vi "ABB Select pages.vi"(7 "Page Names":string[](array[string]), 9 "Report in":string, 10 "Page ends":i32[](array[numeric]), 11 "Page select":bool[](array[boolean])) -> (1 "Report out":string, 2 "Page names out":string[](array[string]), 4 "Pages out":string[](array[string]))   [LabVIEW 2017]
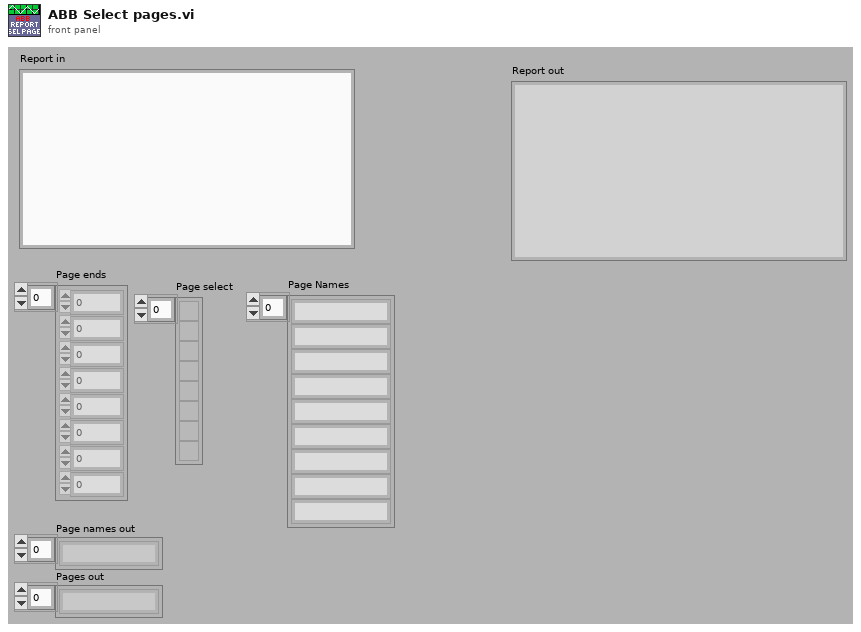
[diagram p1: front panel]
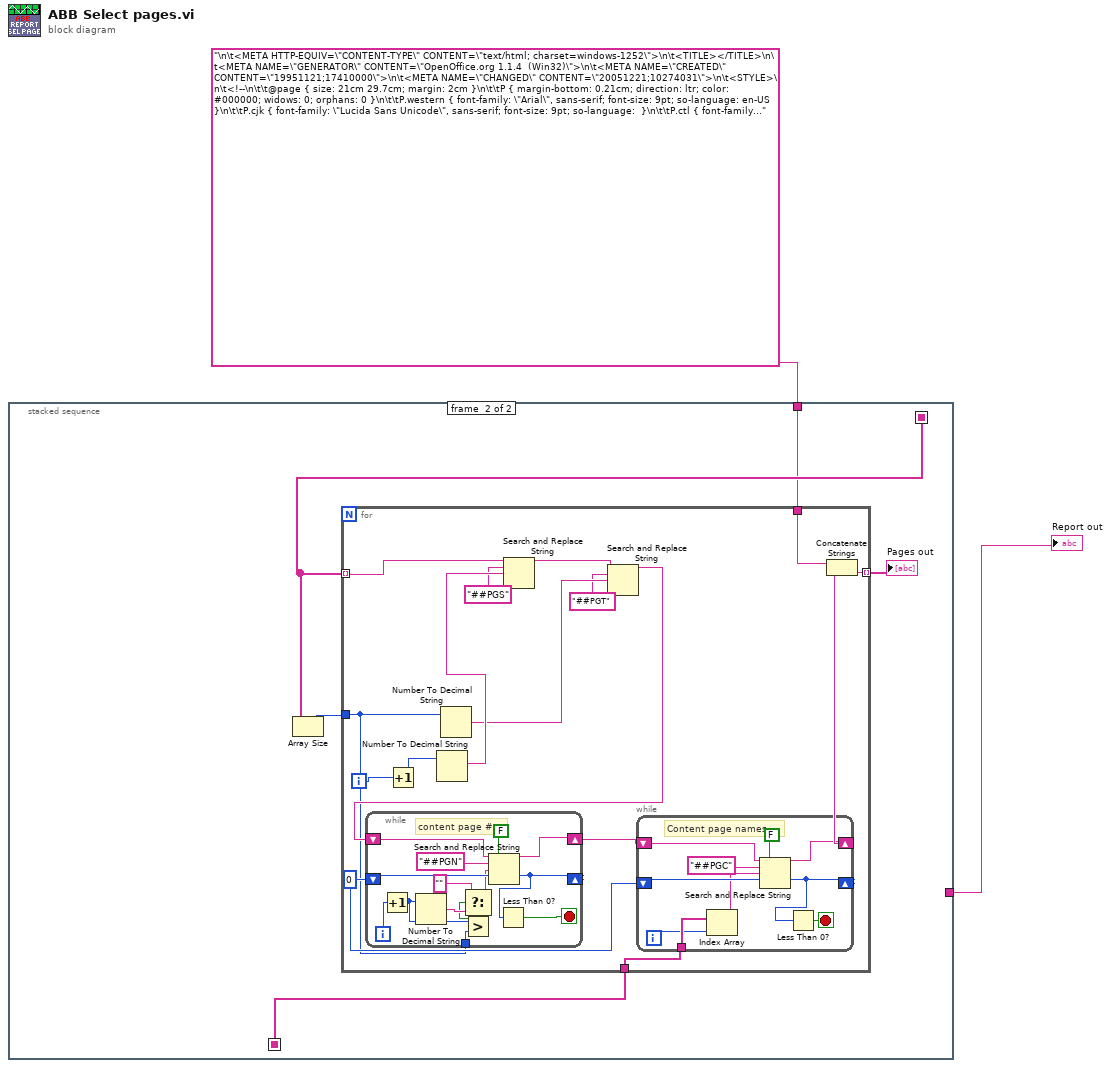
[diagram p0: block diagram]
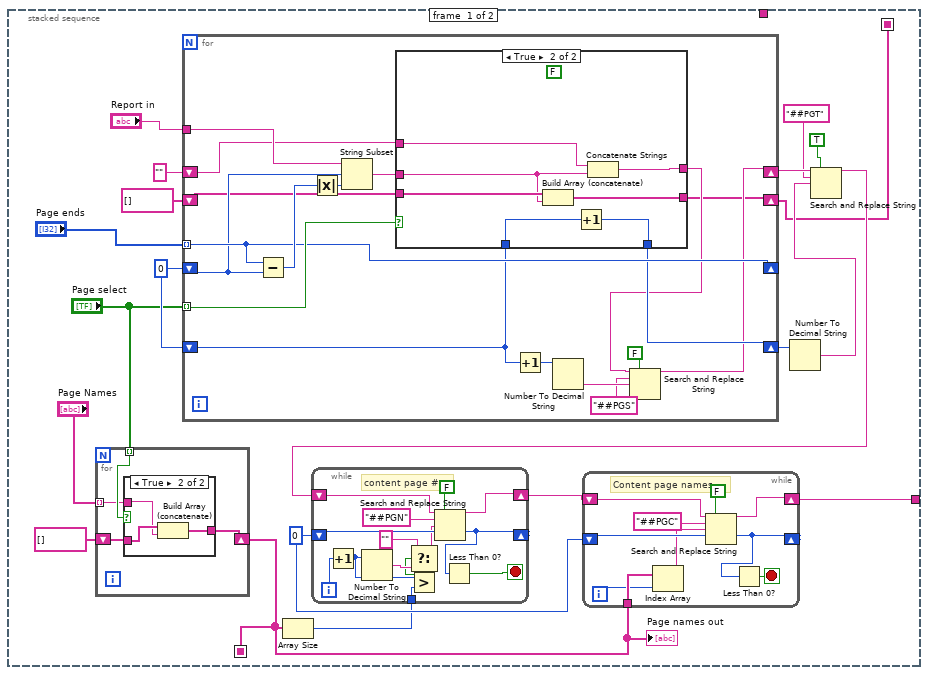
[diagram p2: hidden frame]
diagram:
  n1 = stacked-sequence {
    seq-local: [w4 _] -> [_ w87]
    seq-local: [w3 _] -> [_ w84]
    tunnel: [w11 _] -> w2
    tunnel: "\n\t<META HTTP-EQUIV=\"CONTENT-TYPE\" CONTENT=\"text/html; charset=windows-1252\">\n\t<TITLE></TITLE>\n\t<META NAME=\"GENERATOR\" CONTENT=\"OpenOffice.org 1.1.4  (Win32)\">\n\t<META NAME=\"CREATED\" CONTENT=\"19951121;17410000\">\n\t<META NAME=\"CHANGED\" CONTENT=\"20051221;10274031\">\n\t<STYLE>\n\t<!--\n\t\t@page { size: 21cm 29.7cm; margin: 2cm }\n\t\tP { margin-bottom: 0.21cm; direction: ltr; color: #000000; widows: 0; orphans: 0 }\n\t\tP.western { font-family: \"Arial\", sans-serif; font-size: 9pt; so-language: en-US }\n\t\tP.cjk { font-family: \"Lucida Sans Unicode\", sans-serif; font-size: 9pt; so-language:  }\n\t\tP.ctl { font-family: \"Times New Roman\", serif; font-size: 12pt; so-language:  }\n\t\tP.ww-table-contents-western { font-family: \"Arial\", sans-serif; font-size: 9pt; so-language: en-US }\n\t\tP.ww-table-contents-cjk { font-family: \"Lucida Sans Unicode\", sans-serif; font-size: 9pt; so-language:  }\n\t\tP.ww-table-contents-ctl { font-family: \"Times New Roman\", serif; font-size: 12pt; so-language:  }\n\t-->\n\t</STYLE>\n</HEAD>\n<BODY LANG=\"en-GB\" TEXT=\"#000000\" DIR=\"LTR\">\n<P LANG=\"en-US\" CLASS=\"western\" STYLE=\"margin-bottom: 0cm\"" -> [_ w83]
    frame #0 {
      w12 = 0 ("offset past replacement")
      w19 = 0 ("Numeric")
      n2 = for {
        tunnel: "Page select" -> [w26] mode=indexing
        tunnel: "Page Names" -> [w25] mode=indexing
        shift-right: [w23] -> w3
        shift-left: string[] [] -> [w24]
        n3 = case shown="True" w26 {
          tunnel: w25 -> [_ w29]
          tunnel: w24 -> [w27 w30]
          tunnel: [w27 w28] -> w23
          frame False {
          }
          frame True {
            n4 = Build Array (concatenate)(w30, w29) -> (w28:string[])
          }
        }
      }
      "Page names out" <- w3
      n5 = for {
        shift-right: [w64] -> w18
        shift-left: "" -> [w67]
        tunnel: "Page ends" -> [w70] mode=indexing
        tunnel: "Page select" -> [w72] mode=indexing
        shift-right: [w70] -> _
        shift-left: w19 -> [w66]
        tunnel: "Report in" -> [w68]
        shift-right: [w65] -> w16
        shift-left: w19 -> [w61]
        shift-right: [w55] -> w4
        shift-left: string[] [] -> [w56]
        n6 = Subtract(x=w70, y=w66) -> (x-y=w71:i32)
        n7 = Absolute Value(x=w71) -> (abs(x)=w57:i32)
        n8 = String Subset(string=w68, offset (0)=w66, length (rest)=w57) -> (substring=w69:string)
        n9 = case shown="True" w72 {
          tunnel: w67 -> [w75 w82]
          tunnel: w69 -> [_ w76]
          tunnel: [w75 w81] -> w63
          tunnel: w61 -> [w74 w80]
          tunnel: [w74 w79] -> w65
          tunnel: w56 -> [w73 w78]
          tunnel: [w73 w77] -> w55
          frame False {
          }
          frame True {
            (unwired) FALSE ("replace all? (F)")
            n10 = Build Array (concatenate)(w78, w76) -> (w77:string[])
            n11 = Increment(x=w80) -> (x+1=w79:i32)
            n12 = Concatenate Strings(w82, w76) -> (w81:string)
          }
        }
        n13 = Increment(x=w61) -> (x+1=w60:i32)
        n14 = Number To Decimal String(number=w60) -> (decimal integer string=w59:string)  [unwired: 1 in]
        n15 = Search and Replace String(replace all?=FALSE ("replace all? (F)"), input string=w63, search string="##PGS", replace string=w59) -> (result string=w64:string)  [unwired: 4 in, 3 out]
      }
      n16 = Array Size(array=w3) -> (size(s)=w6:i32)
      n17 = Number To Decimal String(number=w16) -> (decimal integer string=w15:string)  [unwired: 1 in]
      n18 = Search and Replace String(replace all?=TRUE ("replace all? (F)"), input string=w18, search string="##PGT", replace string=w15) -> (result string=w10:string)  [unwired: 4 in, 3 out]
      n19 = while {
        shift-right: [w52] -> w13
        shift-left: w10 -> [w54]
        shift-right: [w49] -> _
        shift-left: w12 -> [w51]
        tunnel: w6 -> [w46]
        i -> [w48]
        stop <- w45 stop-if-true
        # "content page #s"
        n20 = Increment(x=w48) -> (x+1=w47:i32)
        n21 = Number To Decimal String(number=w47) -> (decimal integer string=w44:string)  [unwired: 1 in]
        n22 = Greater?(x=w47, y=w46) -> (0:w42:bool)
        n23 = Select(t="", s=w42, f=w44) -> (s? t:f=w41:string)
        n24 = Search and Replace String(replace all?=FALSE ("replace all? (F)"), input string=w54, search string="##PGN", replace string=w41, offset=w51) -> (result string=w52:string, offset past replacement=w49:i32)  [unwired: 3 in, 2 out]
        n25 = Less Than 0?(x=w49) -> (x < 0?=w45:bool)
      }
      n26 = while {
        shift-right: [w38] -> w11
        shift-left: w13 -> [w40]
        shift-right: [w34] -> _
        shift-left: w12 -> [w37]
        tunnel: w3 -> [w33]
        i -> [w32]
        stop <- w35 stop-if-true
        # "Content page names"
        n27 = Index Array(array=w33, index=w32) -> (element=w31:string)
        n28 = Search and Replace String(replace all?=FALSE ("replace all? (F)"), input string=w40, search string="##PGC", replace string=w31, offset=w37) -> (result string=w38:string, offset past replacement=w34:i32)  [unwired: 3 in, 2 out]
        n29 = Less Than 0?(x=w34) -> (x < 0?=w35:bool)
      }
    }
    frame #1 {
      n30 = Array Size(array=w87) -> (size(s)=w86:i32)
      n31 = for {
        tunnel: w87 -> [w101] mode=indexing
        tunnel: w86 -> [w90]
        tunnel: [w89] -> w85 mode=indexing
        tunnel: w84 -> [w91]
        tunnel: w83 -> [w88]
        i -> [w103]
        w92 = 0 ("offset past replacement")
        n32 = Increment(x=w103) -> (x+1=w102:i32)
        n33 = Number To Decimal String(number=w102) -> (decimal integer string=w100:string)  [unwired: 1 in]
        n34 = Number To Decimal String(number=w90) -> (decimal integer string=w98:string)  [unwired: 1 in]
        n35 = Search and Replace String(input string=w101, search string="##PGS", replace string=w100) -> (result string=w99:string)  [unwired: 5 in, 3 out]
        n36 = Search and Replace String(input string=w99, search string="##PGT", replace string=w98) -> (result string=w94:string)  [unwired: 5 in, 3 out]
        n37 = while {
          shift-right: [w125] -> w95
          shift-left: w94 -> [w127]
          shift-right: [w122] -> _
          shift-left: w92 -> [w124]
          tunnel: w90 -> [w119]
          i -> [w121]
          stop <- w118 stop-if-true
          # "content page #s"
          n38 = Increment(x=w121) -> (x+1=w120:i32)
          n39 = Number To Decimal String(number=w120) -> (decimal integer string=w117:string)  [unwired: 1 in]
          n40 = Greater?(x=w120, y=w119) -> (0:w115:bool)
          n41 = Select(t="", s=w115, f=w117) -> (s? t:f=w114:string)
          n42 = Search and Replace String(replace all?=FALSE ("replace all? (F)"), input string=w127, search string="##PGN", replace string=w114, offset=w124) -> (result string=w125:string, offset past replacement=w122:i32)  [unwired: 3 in, 2 out]
          n43 = Less Than 0?(x=w122) -> (x < 0?=w118:bool)
        }
        n44 = while {
          shift-right: [w111] -> w93
          shift-left: w95 -> [w113]
          shift-right: [w107] -> _
          shift-left: w92 -> [w110]
          tunnel: w91 -> [w106]
          i -> [w105]
          stop <- w108 stop-if-true
          # "Content page names"
          n45 = Index Array(array=w106, index=w105) -> (element=w104:string)
          n46 = Search and Replace String(replace all?=FALSE ("replace all? (F)"), input string=w113, search string="##PGC", replace string=w104, offset=w110) -> (result string=w111:string, offset past replacement=w107:i32)  [unwired: 3 in, 2 out]
          n47 = Less Than 0?(x=w107) -> (x < 0?=w108:bool)
        }
        n48 = Concatenate Strings(w88, w93) -> (w89:string)
      }
      "Pages out" <- w85
    }
  }
  "Report out" <- w2
